vi "Do.vi"(8 "error in (no error)":errorcluster, 10 "Actor in":refnum<class "Actor.lvclass">, 11 "Go to IDLE Msg":refnum<class "Go to IDLE Msg.lvclass">) -> (0 "error out":errorcluster, 2 "Actor out":refnum<class "Actor.lvclass">)   [LabVIEW 2021, in "Chef States.lvlib" / "Go to IDLE Msg.lvclass"]
doc: "This VI delivers the message to the actor by calling the appropriate method(s) on the actor."
uses:
  Go to IDLE Msg.lvclass
  Go to IDLE Msg.lvclass/Go to IDLE Msg.ctl
  9ef47adc-f318-494c-9b8b-6df3216d6863.vi
  Chef State/Chef State.lvclass
  <vilib>/ActorFramework/Actor/Actor.lvclass
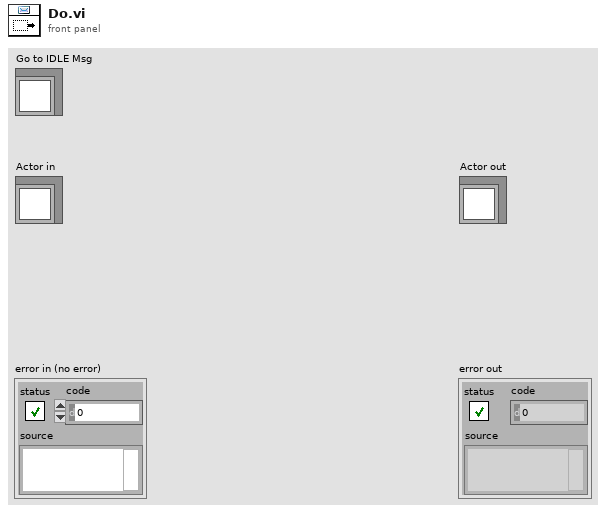
[diagram p1: front panel]
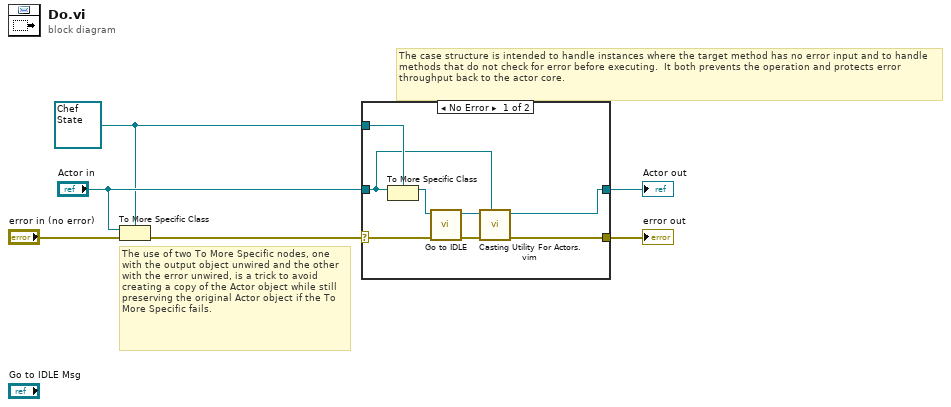
[diagram p0: block diagram]
diagram:
  w1 = refnum<class "Chef State.lvclass"> refnum ("Actor in")
  # "The use of two To More Specific nodes, one with the output object unwired and the other with the error unwired, is a trick to avoid creating a copy of the Actor object while still preserving the original Actor object if the To More Specific fails."
  # "The case structure is intended to handle instances where the target method has no error input and to handle methods that do not check for error before executing.  It both prevents the operation and protects error throughput back to the actor core."
  n1 = To More Specific Class(target class=w1, reference="Actor in", error in="error in (no error)") -> (error out=w5:errorcluster)  [unwired: 1 out]
  n2 = case shown="No Error" w5 {
    selector: w5 -> [w14 w16]
    tunnel: [w10 w16] -> w4
    tunnel: [w11 w15] -> w3
    tunnel: "Actor in" -> [w12 w15]
    tunnel: w1 -> [w13 _]
    frame No Error {
      n3 = To More Specific Class(target class=w13, reference=w12) -> (specific class reference=w8:refnum<class "Chef State.lvclass">)  [unwired: 1 in, 1 out]
      n4 = call-dynamic "Go to IDLE.vi"("error in (no error)"=w14, "Chef State in"=w8) -> ("error out"=w9:errorcluster, "State Actor.lvclass"=w7:refnum<class "State Actor.lvclass">)  [unwired: 8 in]
      n5 = call "Casting Utility For Actors.vim"("type"=w12, "error in (no error)"=w9, "Actor in"=w7) -> ("error out"=w10:errorcluster, "Actor out"=w11:refnum<class "Actor.lvclass">)  [unwired: 7 in]
    }
    frame Error {
      # "If type check fails, pass the original object out again."
    }
  }
  "error out" <- w4
  "Actor out" <- w3
